vi "LoggingLoop.vi"(8 "Error In":errorcluster, 11 "Message Queues":T1) -> (0 "Error Out":errorcluster)   [LabVIEW 2017, in "Server.lvlib" / "Logging.lvlib"]
doc: "This Loop accepts \"Log\"-Messages with LogData.ctl as Datatype. It then logs the Type of Message, the Message Data and the Timestamp of the message to a tdms-file."
uses:
  Logging.lvlib
  Message Queue/CommReferences.ctl
  Message Queue/MessageCluster.ctl
  LogData.ctl
  <vilib>/Utility/error.llb/Error Cluster From Error Code.vi
  SubVIs/Globals.vi
  <vilib>/ErrorRing/Error Ring.xnode
  Message Queue/Message Queue.lvlib
  Server.lvlib
  ErrorLogger/ErrorLogger.lvlib
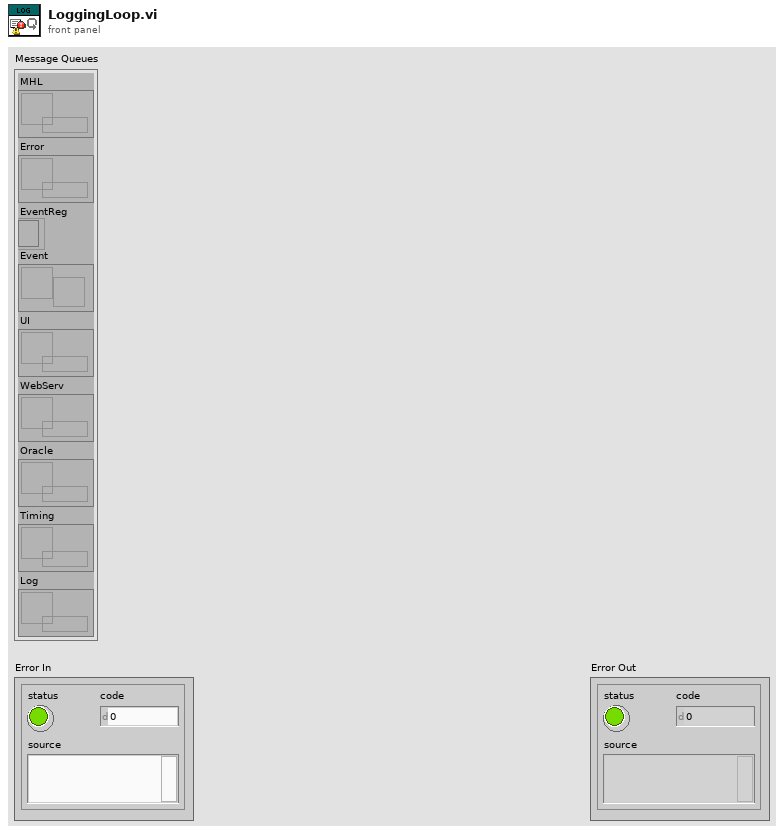
[diagram p1: front panel]
types:
  T1 = typedef "Server.lvlib/Message Queue.lvlib/CommReferences.ctl" = cluster{"MHL":refnum<queue>, "Error":refnum<queue>, "EventReg":refnum<event-registration>, "Event":refnum<user-event>, "UI":refnum<queue>, "WebServ":refnum<queue>, "Oracle":refnum<queue>, "Timing":refnum<queue>, "Log":refnum<queue>}
  T2 = enum16{"open", "open or create", "create or replace", "create", "open (read-only)"}
  T3 = typedef "Server.lvlib/Logging.lvlib/LogData.ctl" = cluster{"Time":timestamp, "Type":string, "LogText":string}
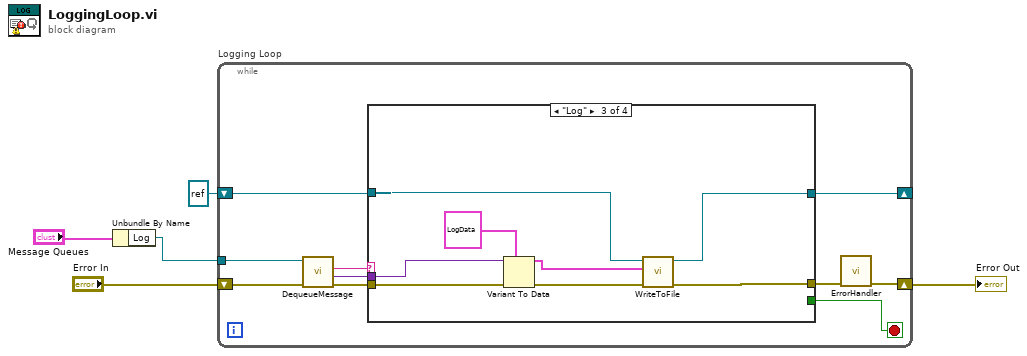
[diagram p0: block diagram]
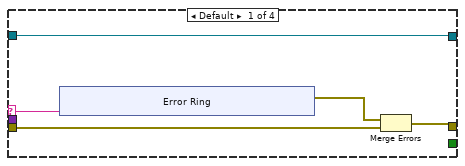
[diagram p2: hidden frame]
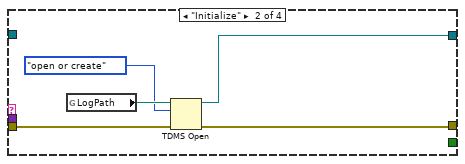
[diagram p3: hidden frame]
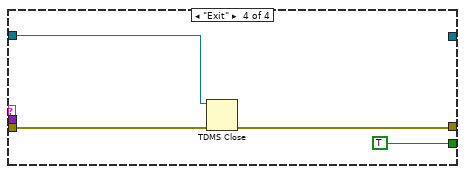
[diagram p4: hidden frame]
diagram:
  n1 = Unbundle By Name("Message Queues") -> ("Log"=w2:refnum<queue>)
  n2 = while "Logging Loop" {
    shift-right: [w6] -> w4
    shift-left: "Error In" -> [w15]
    tunnel: w2 -> [w14]
    shift-right: [w8] -> _
    shift-left: refnum<k34> refnum ("tdms file out") -> [w7]
    stop <- w9 stop-if-true
    n3 = call "DequeueMessage.vi"("error in (no error)"=w15, "Message Queue"=w14) -> ("error out"=w13:errorcluster, "Message Data"=w10:variant, "Message"=w11:string)  [unwired: 5 in, 2 out]
    n4 = case shown="\"Log\"" w11 {
      selector: w11 -> [w19 _ _ _]
      tunnel: [w18 w30 w36 w42] -> w12
      tunnel: w13 -> [w20 w32 w40 w44]
      tunnel: w10 -> [_ _ w38 _]
      tunnel: [_ _ _ TRUE] -> w9
      tunnel: [w16 w28 w34 _] -> w8
      tunnel: w7 -> [w16 _ w35 w41]
      frame Default {
        n5 = xnode "Error Ring"("parameter 0"=w19) -> ("error out"=w17:errorcluster)
        n6 = Merge Errors(w17, w20) -> (w18:errorcluster)
      }
      frame "Initialize" {
        n7 = global read "Globals.vi" "LogPath"() -> (w31:path)
        n8 = TDMS Open(8:w32, 10:T2."open or create" ("operation (0:open)"), 11:w31) -> (0:w30:errorcluster, 3:w28:refnum<k34>)  [unwired: 4 in]
      }
      frame "Log" {
        n9 = Variant To Data(error in=w40, type=T3 {"Time"=timestamp(0 s since 1904-01-01), "Type"="", "LogText"=""} ("LogData"), Variant=w38) -> (data=w33:T3, error out=w39:errorcluster)
        n10 = call "WriteToFile.vi"("error in (no error)"=w39, "LogData"=w33, "Refnum in"=w35) -> ("error out"=w36:errorcluster, "Refnum out"=w34:refnum<k34>)  [unwired: 7 in]
      }
      frame "Exit" {
        n11 = TDMS Close(8:w44, 11:w41) -> (0:w42:errorcluster)  [unwired: 1 out]
      }
    }
    n12 = call "ErrorHandler.vi"("error in (no error)"=w12) -> ("error out"=w6:errorcluster)  [unwired: 10 in]
  }
  "Error Out" <- w4
